vi "continuousMoveStage (SubVI).vi"(0 "Home stage":bool, 1 "Stop Stage":bool, 5 "Move stage":bool, 11 "error in (no error)":errorcluster, 12 "Send stage to XYZ [mm]":T2={"Go to X"=-23.0, "Go to Y"=-32.0, "Go to Z"=3.4}, 14 "Axes Speeds [mm/s]":T1={"X Speed"=25.0, "Y Speed"=12.5, "Z Speed"=5.0}) -> (4 "Homed":bool, 6 "Moving":bool, 8 "N moves":i32=2, 10 "XYZ Stage Current Position":T3={"X [-750, 750 mm]"=-22.99388114929199, "Y [-150, 30 mm]"=-32.00124923706055, "Z [-50, 50 mm]"=3.4108}, 15 "Error report":errorcluster)   [LabVIEW 2016]
uses:
  Motion/HomeMultiple.vi
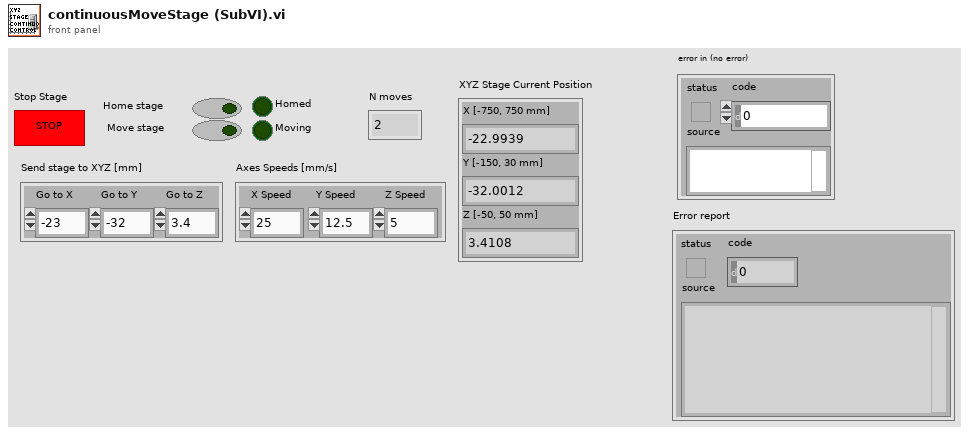
[diagram p1: front panel]
types:
  T1 = cluster{"X Speed":dbl, "Y Speed":dbl, "Z Speed":dbl}
  T2 = cluster{"Go to X":dbl, "Go to Y":dbl, "Go to Z":dbl}
  T3 = cluster{"X [-750, 750 mm]":dbl, "Y [-150, 30 mm]":dbl, "Z [-50, 50 mm]":dbl}
  T4 = cluster{"Program Position Feedback":dbl, "Program Position Feedback 2":dbl, "Program Position Feedback 3":dbl}
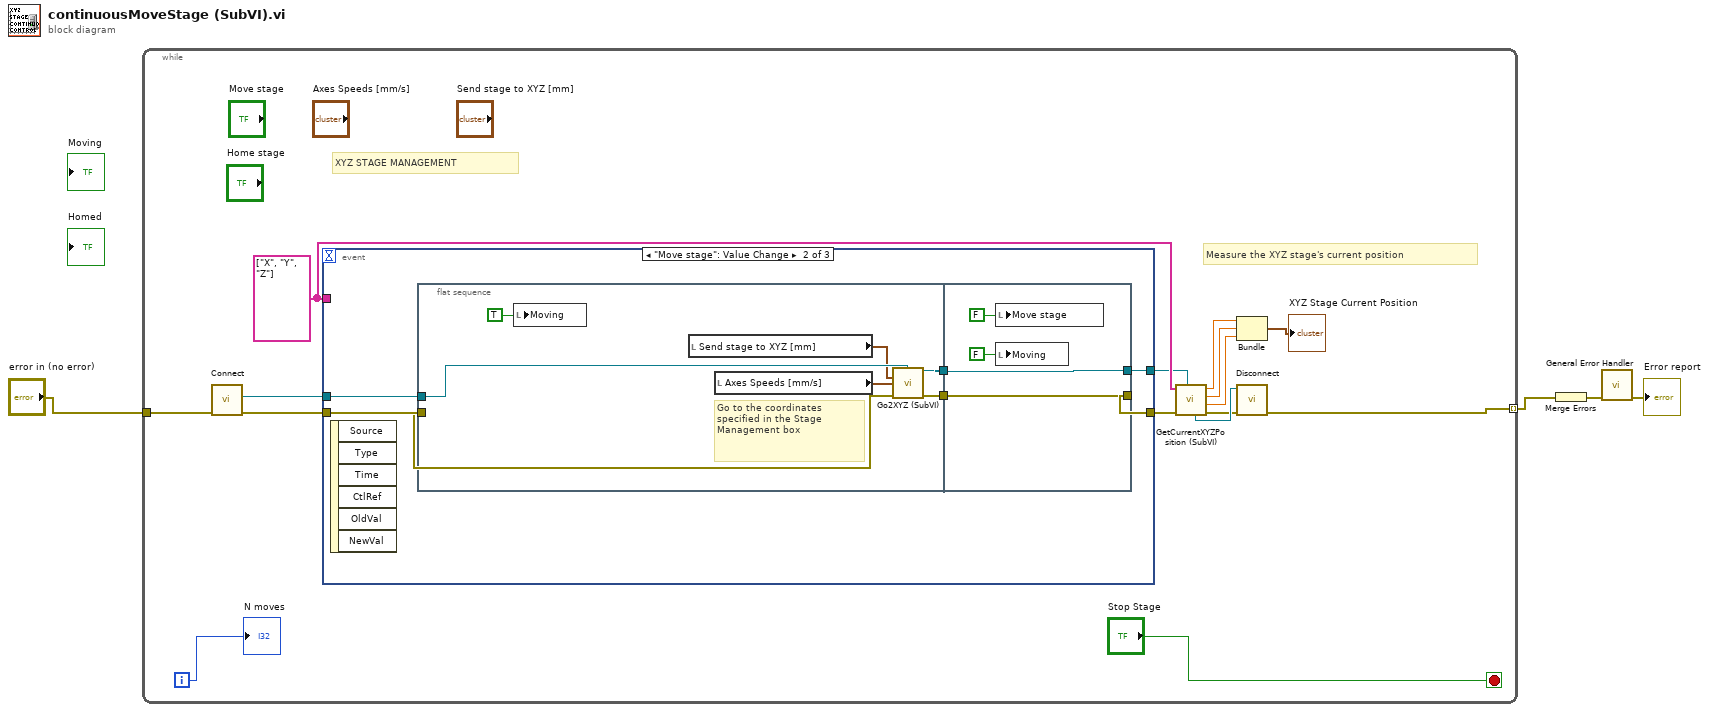
[diagram p0: block diagram]
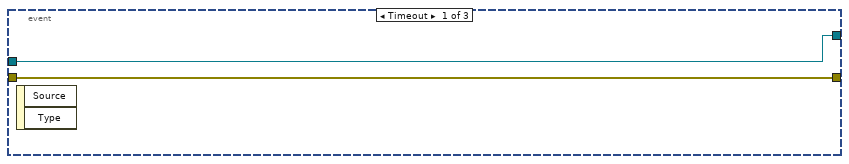
[diagram p2: hidden frame]
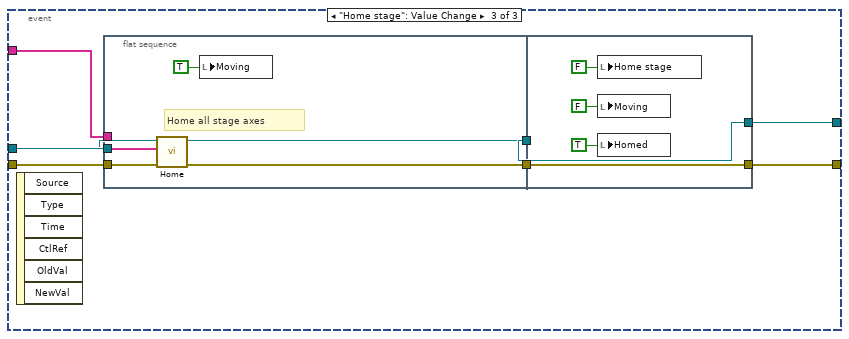
[diagram p3: hidden frame]
diagram:
  n1 = while {
    tunnel: "error in (no error)" -> [w6]
    tunnel: [w5] -> w1 mode=indexing
    i -> [w7]
    stop <- "Stop Stage" stop-if-true
    w11 = string[] ["X", "Y", "Z"] ("Axes Names")
    # "XYZ STAGE MANAGEMENT"
    # "Measure the XYZ stage's current position"
    n2 = call "Connect.vi"("error in (no error)"=w6) -> ("error out"=w18:errorcluster, "controller"=w19:refnum<k24>)  [unwired: 9 in]
    n3 = event shown="[1] \"Move stage\": Value Change" {
      selector: _ -> [_ _ _]
      dyn-events: _ -> [_ _ _]
      timeout: _ -> [_ _ _]
      tunnel: w19 -> [w21 w27 w45]
      tunnel: w18 -> [w20 w24 w44]
      tunnel: [w21 w26 w42] -> w10
      tunnel: [w20 w25 w43] -> w12
      tunnel: w11 -> [_ _ w41]
      event Timeout {
        n4 = event-data() -> ()  [unwired: 1 in, 2 out]
      }
      event "Move stage": Value Change {
        n5 = event-data() -> ()  [unwired: 1 in, 6 out]
        n6 = flat-sequence {
          tunnel: w27 -> [w34]
          tunnel: w24 -> [w31]
          tunnel: [w33] -> w23
          tunnel: [w32] -> w22
          tunnel: [w37] -> w25
          tunnel: [w38] -> w26
          tunnel: w23 -> [w38]
          tunnel: w22 -> [w37]
          frame #0 {
            # "Go to the coordinates\nspecified in the Stage\nManagement box"
            n7 = local write "Moving"(TRUE ("Moving")) -> ()
            n8 = local read "Send stage to XYZ [mm]"() -> (w29:T2)
            n9 = local read "Axes Speeds [mm/s]"() -> (w28:T1)
            n10 = call "Go2XYZ (SubVI).vi"(".NET Refnum in"=w34, "Go to Coordinates"=w29, "Axis Speeds"=w28, "error in (no error)"=w31) -> (".NET Refnum out"=w33:refnum<k24>, "error out"=w32:errorcluster)  [unwired: 8 in, 2 out]
          }
          frame #1 {
            n11 = local write "Move stage"(FALSE ("Move stage")) -> ()
            n12 = local write "Moving"(FALSE ("Moving")) -> ()
          }
        }
      }
      event "Home stage": Value Change {
        n13 = event-data() -> ()  [unwired: 1 in, 6 out]
        n14 = flat-sequence {
          tunnel: w45 -> [w51]
          tunnel: w44 -> [w50]
          tunnel: w41 -> [w47]
          tunnel: [w49] -> w40
          tunnel: [w48] -> w39
          tunnel: [w55] -> w42
          tunnel: [w56] -> w43
          tunnel: w40 -> [w56]
          tunnel: w39 -> [w55]
          frame #0 {
            # "Home all stage axes"
            n15 = call-poly "Home.vi"("error in (no error)"=w50, "axis names"=w47, "controller in"=w51) -> ("error out"=w49:errorcluster, "controller out"=w48:refnum<k24>)  [unwired: 7 in]
            n16 = local write "Moving"(TRUE ("Moving")) -> ()
          }
          frame #1 {
            n17 = local write "Home stage"(FALSE ("Home stage")) -> ()
            n18 = local write "Moving"(FALSE ("Moving")) -> ()
            n19 = local write "Homed"(TRUE ("Homed")) -> ()
          }
        }
      }
    }
    n20 = call "GetCurrentXYZPosition (SubVI).vi"(".NET Refnum in - Device"=w10, "error in (no error)"=w12, "Axes Names"=w11) -> ("error out"=w9:errorcluster, "Program Position Feedback 3"=w17:dbl, "Program Position Feedback 2"=w16:dbl, "Program Position Feedback"=w15:dbl, ".NET Refnum out  - Device"=w14:refnum<k24>)  [unwired: 3 in]
    n21 = Bundle("Program Position Feedback"=w15, "Program Position Feedback 2"=w16, "Program Position Feedback 3"=w17) -> (→"XYZ Stage Current Position":T4)  [unwired: 1 in]
    n22 = call "Disconnect.vi"("error in (no error)"=w9, "controller"=w14) -> ("error out"=w5:errorcluster)  [unwired: 9 in]
    "N moves" <- w7
  }
  n23 = Merge Errors(w1) -> (w3:errorcluster)
  n24 = call <vilib>:"General Error Handler.vi"("error in (no error)"=w3) -> ("error out"=→"Error report":errorcluster)  [unwired: 2 in, 12 out]
